vi "Example4.vi"() -> ()   [LabVIEW 2019]
uses:
  source code/Container/dotNET Container/dotNET Container.lvclass
  D:/Modern Labs/semi-val-fw-prototype/prototypes/mdi-hosted-app/src/MDI/source code/Container/Container base/Container base.lvclass
  source code/Document/LV Doc/Child/LV DEV/LV DEV.lvclass
  D:/Modern Labs/semi-val-fw-prototype/prototypes/mdi-hosted-app/src/MDI/source code/Document/Document base/Document.lvclass
  source code/MDI Library/Public/Create.vi
  source code/Document/LV Doc/Child/LV DEV/public/LV Dev Doc - Instantiate with Path.vi
  source code/MDI Library/Public/Add.vi
  source code/MDI Library/Public/Show.vi
  source code/MDI Library/Public/Tile.vi
  source code/MDI Library/Public/Cascade.vi
  source code/MDI Library/Public/Dock.vi
  source code/MDI Library/Public/Remove.vi
  source code/Document/Document base/Document.lvclass
  source code/MDI Library/LV MDI.lvclass
  D:/Modern Labs/semi-val-fw-prototype/prototypes/mdi-hosted-app/src/MDI/source code/Document/LV Doc/LV Doc.lvclass
  System.Windows.Forms
panel:
  in  "Dock?":bool
  in  "LabVIEW Version":u16(ring) items=["LabVIEW 2019", "LabVIEW 2018", "LabVIEW 2016"]
  in  "Cascade":bool
  in  "Tile":bool
  in  "Stop":bool
  in  "Show":bool
  in  "LV Doc Path":path=path "D:/Namratha/Study/Hosted Application/MDI/MDI/example/Example1/Plugin/Waveform.vi"
  in  "Panel Reference":refnum<k24>(container)
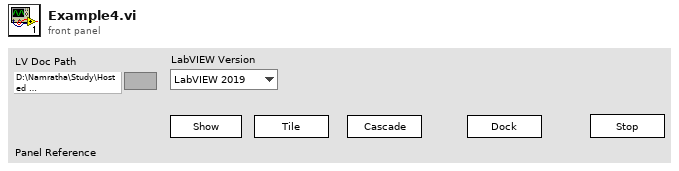
[diagram p1: front panel]
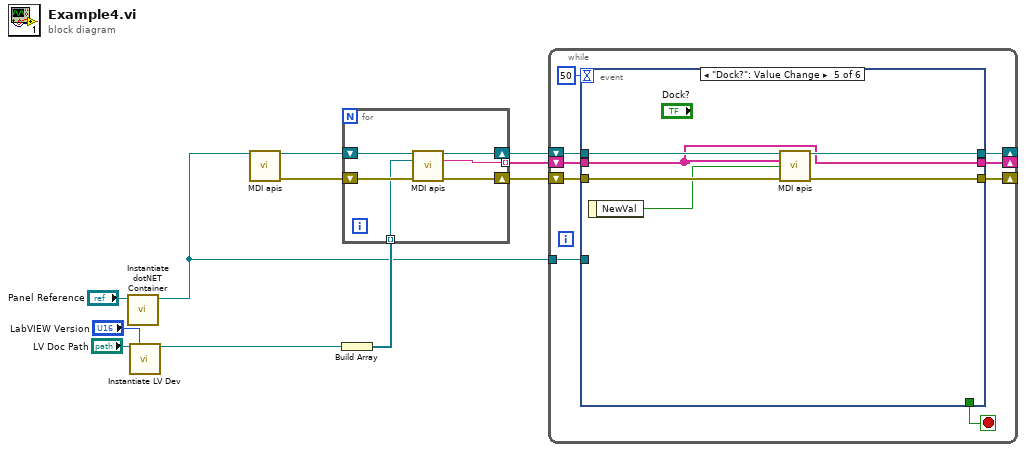
[diagram p0: block diagram]
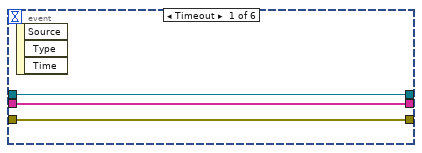
[diagram p2: hidden frame]
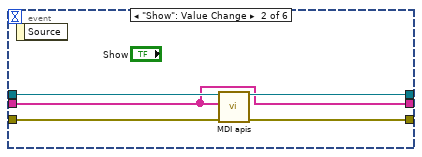
[diagram p3: hidden frame]
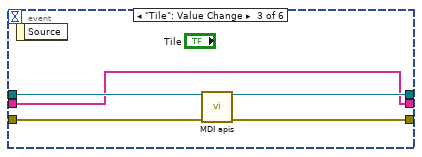
[diagram p4: hidden frame]
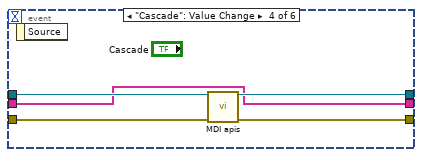
[diagram p5: hidden frame]
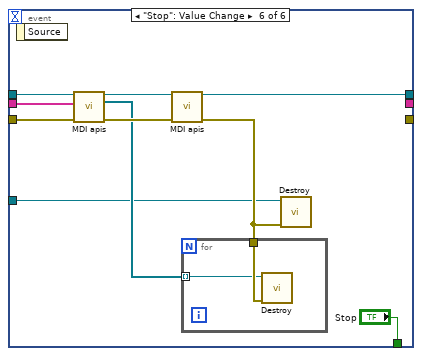
[diagram p6: hidden frame]
diagram:
  n1 = call "Instantiate dotNET Container.vi"("Panel Reference"="Panel Reference") -> ("dotNET Container out"=w2:refnum<class "dotNET Container.lvclass">)  [unwired: 9 in, 1 out]
  n2 = call-poly "Instantiate LV Dev.vi"("LV Doc Path"="LV Doc Path", "LabVIEW Version"="LabVIEW Version") -> ("LV DEV"=w7:refnum<class "LV DEV.lvclass">)  [unwired: 12 in, 1 out]
  n3 = call-poly "MDI apis.vi"("Container"=w2) -> ("LV MDI"=w11:refnum<class "LV MDI.lvclass">, "error out"=w10:errorcluster)  [unwired: 13 in]
  n4 = Build Array(w7) -> (w9:refnum<class "LV DEV.lvclass">[])
  n5 = for {
    shift-right: [w15] -> w4
    shift-left: w11 -> [w17]
    shift-right: [w14] -> w5
    shift-left: w10 -> [w16]
    tunnel: w9 -> [w13] mode=indexing
    tunnel: [w12] -> w3 mode=indexing
    n6 = call-poly "MDI apis.vi"("LV MDI.lvclass"=w17, "Document class"=w13, "error in (no error)"=w16) -> ("LV MDI.lvclass"=w15:refnum<class "LV MDI.lvclass">, "Doc UID"=w12:string, "error out"=w14:errorcluster)  [unwired: 10 in]
  }
  n7 = while {
    shift-right: [w23] -> _
    shift-left: w5 -> [w24]
    shift-right: [w21] -> _
    shift-left: w4 -> [w22]
    tunnel: w2 -> [w19]
    shift-right: [w18] -> _
    shift-left: w3 -> [w20]
    stop <- w25 stop-if-true
    n8 = event shown="[4] \"Dock?\": Value Change" {
      selector: _ -> [_ _ _ _ _ _]
      dyn-events: _ -> [_ _ _ _ _ _]
      timeout: 50 -> [_ _ _ _ _ _]
      tunnel: [_ _ _ _ _ "Stop"] -> w25
      tunnel: w24 -> [w29 w34 w38 w42 w48 w55]
      tunnel: [w29 w33 w37 w41 w47 _] -> w23
      tunnel: w22 -> [w28 w32 w39 w44 w50 w54]
      tunnel: [w28 w31 w36 w43 w49 w53] -> w21
      tunnel: w20 -> [w27 w30 w35 w40 w45 w51]
      tunnel: w19 -> [_ _ _ _ _ w52]
      tunnel: [w27 w30 w35 w40 w45 _] -> w18
      event Timeout {
        n9 = event-data() -> ()  [unwired: 1 in, 3 out]
      }
      event "Show": Value Change {
        n10 = event-data() -> ()  [unwired: 1 in, 1 out]
        n11 = call-poly "MDI apis.vi"("LV MDI in"=w32, "Doc UID[]"=w30, "error in (no error)"=w34) -> ("LV MDI out"=w31:refnum<class "LV MDI.lvclass">, "error out"=w33:errorcluster)  [unwired: 11 in]
      }
      event "Tile": Value Change {
        n12 = event-data() -> ()  [unwired: 1 in, 1 out]
        n13 = call-poly "MDI apis.vi"("LV MDI.lvclass"=w39, "error in (no error)"=w38) -> ("LV MDI.lvclass"=w36:refnum<class "LV MDI.lvclass">, "error out"=w37:errorcluster)  [unwired: 12 in]
      }
      event "Cascade": Value Change {
        n14 = event-data() -> ()  [unwired: 1 in, 1 out]
        n15 = call-poly "MDI apis.vi"("LV MDI in"=w44, "error in (no error)"=w42) -> ("LV MDI out"=w43:refnum<class "LV MDI.lvclass">, "error out"=w41:errorcluster)  [unwired: 12 in]
      }
      event "Dock?": Value Change {
        n16 = event-data() -> ("NewVal"=w46:bool)  [unwired: 1 in]
        n17 = call-poly "MDI apis.vi"("LV MDI.lvclass"=w50, "Doc UID[]"=w45, "Undock?"=w46, "error in (no error)"=w48) -> ("LV MDI.lvclass"=w49:refnum<class "LV MDI.lvclass">, "error out"=w47:errorcluster)  [unwired: 10 in]
      }
      event "Stop": Value Change {
        n18 = event-data() -> ()  [unwired: 1 in, 1 out]
        n19 = call-poly "MDI apis.vi"("LV MDI in"=w54, "Doc UID[]"=w51, "error in (no error)"=w55) -> ("LV MDI out"=w58:refnum<class "LV MDI.lvclass">, "Doc obj[]"=w56:refnum<class "Document.lvclass">[], "error out"=w57:errorcluster)  [unwired: 10 in]
        n20 = call-poly "MDI apis.vi"("LV MDI in"=w58, "error in (no error)"=w57) -> ("LV MDI out"=w53:refnum<class "LV MDI.lvclass">, "error out"=w59:errorcluster)  [unwired: 12 in]
        n21 = for {
          tunnel: w59 -> [w62]
          tunnel: w56 -> [w61] mode=indexing
          n22 = call-dynamic "Destroy.vi"("error in (no error)"=w62, "Document in"=w61) -> ()  [unwired: 8 in, 2 out]
        }
        n23 = call-dynamic "Destroy.vi"("error in (no error)"=w59, "dotNET Container in"=w52) -> ()  [unwired: 8 in, 2 out]
      }
    }
  }
